vi "Try 2.vi"() -> ()   [LabVIEW 2014]
uses:
  Arduino TFT.lvlib
panel:
  out "Error Out":errorcluster
  in  "Error In":errorcluster
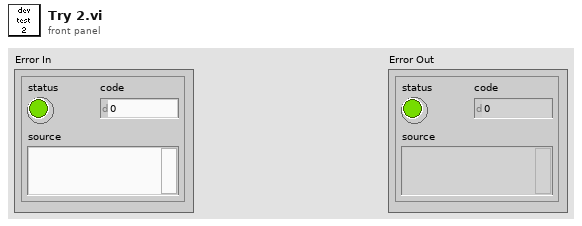
[diagram p1: front panel]
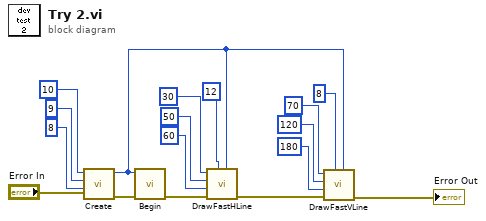
[diagram p0: block diagram]
diagram:
  n1 = call "Create.vi"("Error In"="Error In", "rst"=u8 8 ("cs"), "rs"=u8 9 ("cs"), "cs"=u8 10) -> ("Error Out"=w16:errorcluster, "Instance"=w5:u32)  [unwired: 4 in]
  n2 = call "Begin.vi"("Error In"=w16, "Instance"=w5) -> ("Error Out"=w12:errorcluster)  [unwired: 8 in]
  n3 = call "DrawFastHLine.vi"("Instance"=w5, "color"=u8 12 ("x"), "Error In"=w12, "width"=u8 60 ("x"), "y"=u8 50 ("x"), "x"=u8 30) -> ("Error Out"=w11:errorcluster)  [unwired: 5 in]
  n4 = call "DrawFastVLine.vi"("Instance"=w5, "color"=u8 8 ("x"), "Error In"=w11, "height"=u8 180 ("x"), "y"=u8 120 ("x"), "x"=u8 70) -> ("Error Out"=→"Error Out":errorcluster)  [unwired: 5 in]
